vi "ICM Update Date and Time.vi"(8 "error in (no error)":errorcluster, 10 "ICM File In":path) -> (0 "error out":errorcluster, 3 "output cluster":T1 {"Time" format="%<%H:%M:%S>t"; "Date" format="%<%Y/%m/%d>T"; "Version" format="%.1g"})   [LabVIEW 2018]
doc: "ICM Update Date and Time.vi\n\nThis VI is sets the Date and Time of the General Parameters to the current date and time. It is called whenever any module saves configurationd data, or when a streaming data file is started.\n\nInstrument Communication Module Version 1.0\nApril, 2018 Original Code Consulting David Thomson\n www.originalcode.com"
uses:
  Controls/ICM General Parameters.ctl
panel:
  # "The values for these\nparameters are generally\nset by the ICM system and\nneed not be edited directly."
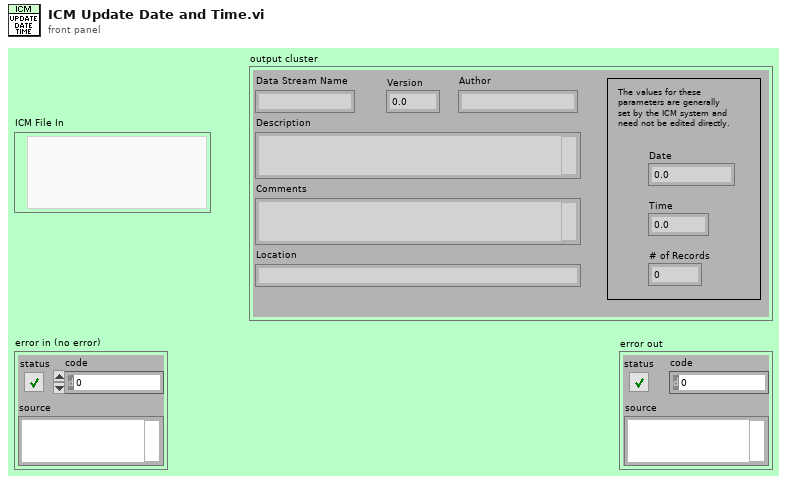
[diagram p1: front panel]
types:
  T1 = typedef "ICM General Parameters.ctl" = cluster{"Data Stream Name":string, "Version":sgl, "Author":string, "Description":string, "Comments":string, "Date":dbl, "Time":dbl, "Location":string, "# of Records":i32}
  T2 = typedef "LVDateTimeRec.ctl" = cluster{"fractional second":dbl, "second":i32, "minute":i32, "hour":i32, "day of month":i32, "month":i32, "year":i32, "day of week":i32, "day of year":i32, "DST":i32}
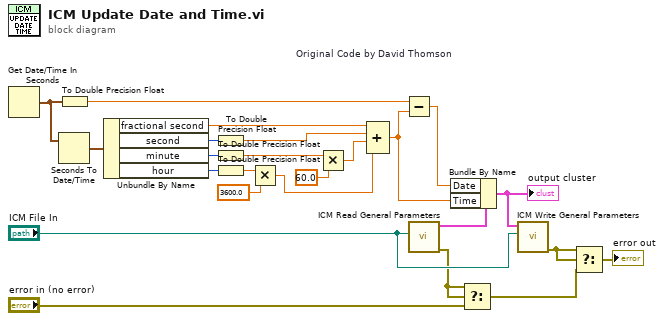
[diagram p0: block diagram]
diagram:
  n1 = Get Date/Time In Seconds() -> (seconds since 1Jan1904=w1:timestamp)
  n2 = Seconds To Date/Time(time stamp (now)=w1) -> (date time rec=w5:T2)  [unwired: 1 in]
  n3 = To Double Precision Float(number=w1) -> (double precision float=w2:dbl)
  n4 = Unbundle By Name "Original Code by David Thomson"(w5) -> ("fractional second"=w16:dbl, "second"=w15:i32, "minute"=w13:i32, "hour"=w12:i32)
  n5 = To Double Precision Float(number=w15) -> (double precision float=w14:dbl)
  n6 = To Double Precision Float(number=w13) -> (double precision float=w11:dbl)
  n7 = To Double Precision Float(number=w12) -> (double precision float=w8:dbl)
  n8 = Multiply(x=w8, y=3600.0) -> (x*y=w7:dbl)
  n9 = Multiply(x=w11, y=60.0) -> (x*y=w10:dbl)
  n10 = Compound Arithmetic op=ADD(w16, w14, w10, w7) -> (w4:dbl)
  n11 = Subtract(x=w2, y=w4) -> (x-y=w3:dbl)
  n12 = call "ICM Read General Parameters.vi"("ICM File In"="ICM File In") -> ("error out"=w18:errorcluster, "ICM General Parameters"=w22:T1)  [unwired: 6 in, 3 out]
  n13 = Bundle By Name(cluster=w22, "Date"=w3, "Time"=w4) -> (w21:T1)
  "output cluster" <- w21
  n14 = Select(t=w18, s=w18, f="error in (no error)") -> (s? t:f=w17:errorcluster)
  n15 = call "ICM Write General Parameters.vi"("ICM File In"="ICM File In", "ICM General Parameters"=w21) -> ("error out"=w24:errorcluster)  [unwired: 9 in]
  n16 = Select(t=w24, s=w24, f=w17) -> (s? t:f=→"error out":errorcluster)
